vi "generate notifiers.vi"(8 "error in (no error)":errorcluster, 11 "Template in":refnum<class "Template.lvclass">) -> (0 "error out":errorcluster, 3 "Template out":refnum<class "Template.lvclass">)   [LabVIEW 2020, in "Template.lvlib" / "Template.lvclass"]
uses:
  Template.lvclass
  typedefs/base actor notifiers.ctl
  Template.lvclass/Template.ctl
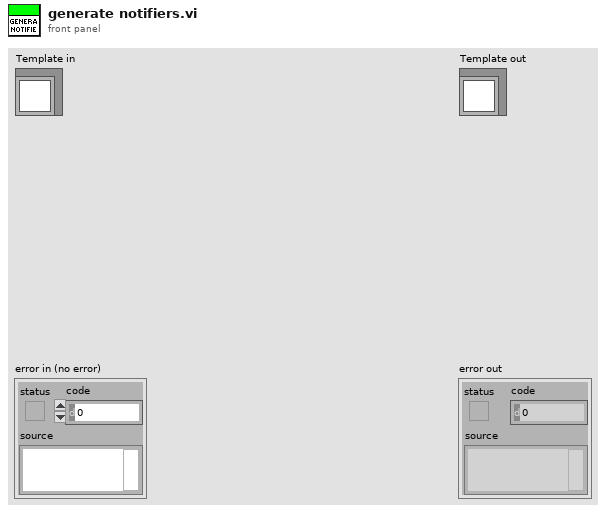
[diagram p1: front panel]
types:
  T1 = typedef "Template.lvlib/Template.lvclass/base actor notifiers.ctl" = cluster{"Stop Actor":refnum<notifier>}
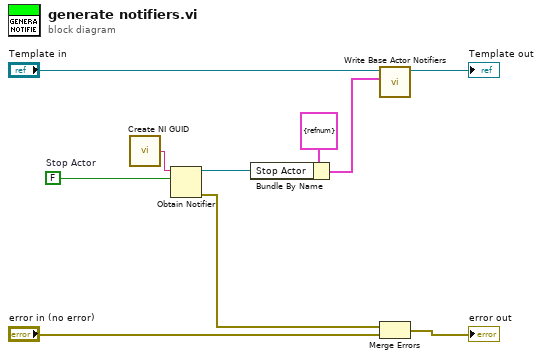
[diagram p0: block diagram]
diagram:
  w6 = FALSE  # Stop Actor
  n1 = call <vilib>:"Create NI GUID.vi"() -> ("NI GUID"=w5:string)
  n2 = Obtain Notifier(name (unnamed)=w5, notification data type=w6) -> (notifier out=w1:refnum<notifier>, error out=w4:errorcluster)  [unwired: 2 in, 1 out]
  n3 = Bundle By Name(cluster=T1 {"Stop Actor"=refnum} ("Base Actor Notifiers"), "Stop Actor"=w1) -> (w2:T1)
  n4 = call "Write Base Actor Notifiers.vi"("Base Actor Notifiers"=w2, "Template in"="Template in") -> ("Template out"=→"Template out":refnum<class "Template.lvclass">)  [unwired: 9 in]
  n5 = Merge Errors(w4, "error in (no error)") -> (→"error out":errorcluster)
